vi "WaitForMessage.vi"(8 "error in (no error)":errorcluster, 9 "timeout in ms (10000)":i32=10000, 11 "STOMP in":refnum<class "STOMP.lvclass">) -> (0 "error out":errorcluster, 1 "timed out?":bool, 2 "message":T1, 3 "STOMP out":refnum<class "STOMP.lvclass">)   [LabVIEW 2017, in "STOMP.lvclass"]
uses:
  STOMP.lvclass
  Typedefs/Type_ServerFrame.ctl
  Typedefs/Type_ServerFrameType.ctl
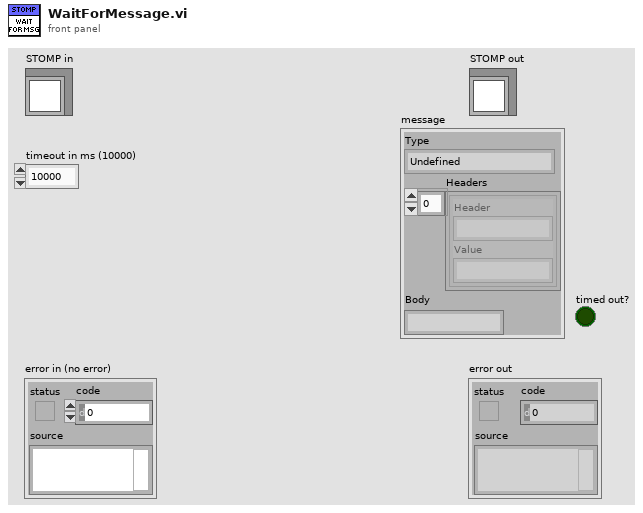
[diagram p1: front panel]
types:
  T1 = typedef "STOMP.lvclass/Type_ServerFrame.ctl" = cluster{"Type":T2, "Headers":cluster{"Header":string, "Value":string}[], "Body":string}
  T2 = typedef "STOMP.lvclass/Type_ServerFrameType.ctl" = enum16{"Undefined", "MESSAGE", "CONNECTED", "RECEIPT", "ERROR"}
  T3 = typedef "STOMP.lvclass/ObjectAttributes.ctl" = cluster{"address":string, "port":u16, "ConnectionRef":refnum<k5>, "messageQueue":refnum<queue>, "receiptQueue":refnum<queue>, "errorQueue":refnum<queue>, "sendQueue":refnum<queue>, "currentReceiptNumber":u64, "currentSubscriptionId":u64, "closeConnection":bool, "activeSubscriptions":T4[]}
  T4 = typedef "STOMP.lvclass/Type_ActiveSubscription.ctl" = cluster{"id":u64, "receipt":bool, "Destination":string, "ack":T5, "headers":T6[]}
  T5 = typedef "STOMP.lvclass/Type_AckHeader.ctl" = enum16{"auto", "client", "client-individual"}
  T6 = typedef "STOMP.lvclass/Type_FrameHeader.ctl" = cluster{"Header":string, "Value":string}
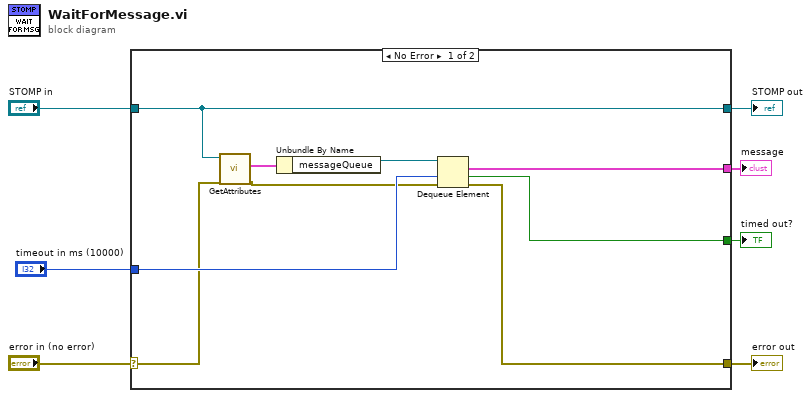
[diagram p0: block diagram]
diagram:
  n1 = case shown="No Error" "error in (no error)" {
    selector: "error in (no error)" -> [w10 w18]
    tunnel: [w9 w18] -> w6
    tunnel: [w13 w17] -> w4
    tunnel: "STOMP in" -> [w13 w17]
    tunnel: "timeout in ms (10000)" -> [w15 _]
    tunnel: [w14 _] -> w2
    tunnel: [w8 _] -> w1
    frame No Error {
      n2 = call-dynamic "GetAttributes.vi"("error in (no error)"=w10, "STOMP in"=w13) -> ("error out"=w11:errorcluster, "attributes"=w12:T3)  [unwired: 7 in, 1 out]
      n3 = Unbundle By Name(w12) -> ("messageQueue"=w16:refnum<queue>)
      n4 = Dequeue Element(queue=w16, timeout in ms (-1)=w15, error in (no error)=w11) -> (element=w14:T1, timed out?=w8:bool, error out=w9:errorcluster)  [unwired: 1 out]
    }
    frame Error {
    }
  }
  "error out" <- w6
  "STOMP out" <- w4
  "message" <- w2
  "timed out?" <- w1
